vi "Run Filter.vi"(8 "error in (no error)":errorcluster, 10 "resource entries in":T1[](array[typedef]) {"FPGA CD Ref" format="%.0x"; "reserver" format="%.0x"}, 11 "OR Filter in":refnum<class "OR Filter.lvclass">) -> (0 "error out":errorcluster, 2 "resource entries out":T1[](array[typedef]) {"FPGA CD Ref" format="%.0x"; "reserver" format="%.0x"})   [LabVIEW 2016, in "FPGA Resource Manager.lvlib" / "OR Filter.lvclass"]
uses:
  OR Filter.lvclass
  Server/resource info.ctl
  <vilib>/NI Veristand/Custom Device API/Custom Device Item Ref.ctl
  OR Filter.lvclass/OR Filter.ctl
  Filter Parent/Filter.lvclass
  <vilib>/NI VeriStand/Custom Device API/Custom Device API.lvlib
  FPGA Resource Manager.lvlib
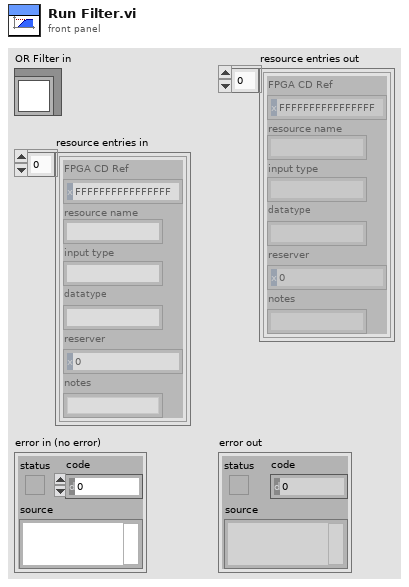
[diagram p1: front panel]
types:
  T1 = typedef "FPGA Resource Manager.lvlib/resource info.ctl" = cluster{"FPGA CD Ref":T2, "resource name":string, "input type":string, "datatype":string, "reserver":T2, "notes":string}
  T2 = typedef "Custom Device API.lvlib/Custom Device Item Ref.ctl" = u64
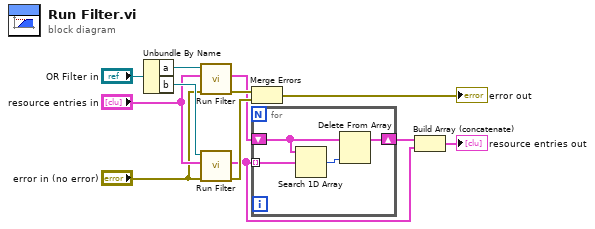
[diagram p0: block diagram]
diagram:
  n1 = Unbundle By Name("OR Filter in") -> ("a"=w11:refnum<class "Filter.lvclass">, "b"=w10:refnum<class "Filter.lvclass">)
  n2 = call-dynamic "Run Filter.vi"("error in (no error)"="error in (no error)", "resource entries in"="resource entries in", "Filter in"=w11) -> ("error out"=w7:errorcluster, "resource entries out"=w4:T1[])  [unwired: 7 in]
  n3 = call-dynamic "Run Filter.vi"("error in (no error)"="error in (no error)", "resource entries in"="resource entries in", "Filter in"=w10) -> ("error out"=w6:errorcluster, "resource entries out"=w2:T1[])  [unwired: 7 in]
  n4 = Merge Errors(w7, w6) -> (→"error out":errorcluster)
  n5 = for {
    tunnel: w2 -> [w16] mode=indexing
    shift-right: [w13] -> w3
    shift-left: w4 -> [w14]
    n6 = Search 1D Array(1D array=w14, element=w16) -> (index of element=w15:i32)  [unwired: 1 in]
    n7 = Delete From Array(array=w14, index=w15) -> (array with subset deleted=w13:T1[])  [unwired: 1 in, 1 out]
  }
  n8 = Build Array (concatenate)(w3, w2) -> (→"resource entries out":T1[])
